vi "xmlParser.vi"(8 "error in (no error)":errorcluster, 10 "XPath Expression":string, 11 "XML File Path":path) -> (0 "error out":errorcluster, 1 "outputArray":string[](array[string]), 2 "outputXML":string, 3 "outputString":string)   [LabVIEW 2018]
uses:
  <vilib>/xml/Close Reference(Node).vi
  <vilib>/xml/NI_XML.lvlib
  <resource>/objmgr/DOMUserDefRef.rc
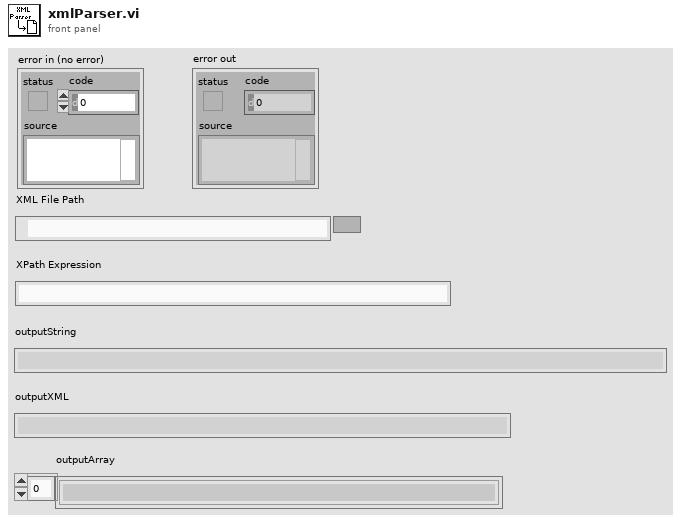
[diagram p1: front panel]
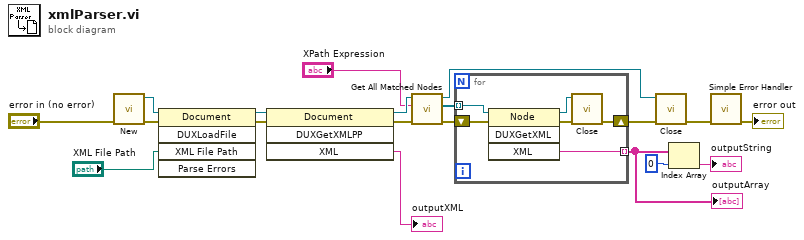
[diagram p0: block diagram]
diagram:
  n1 = call <vilib>:"New.vi"("error in (no error)"="error in (no error)") -> ("error out"=w12:errorcluster, "DOM document out"=w13:refnum<k20>)  [unwired: 7 in]
  n2 = invoke class="Document" method="DUXLoadFile"(reference=w13, error in=w12, "XML File Path"="XML File Path") -> (reference out=w10:refnum<k20>, error out=w11:errorcluster)  [unwired: 2 in, 3 out]
  n3 = invoke class="Document" method="DUXGetXMLPP"(reference=w10, error in=w11) -> (reference out=w14:refnum<k20>, error out=w15:errorcluster, "XML"=→"outputXML":string)  [unwired: 2 in, 1 out]
  n4 = call <vilib>:"Get All Matched Nodes.vi"("error in (no error)"=w15, "XPath expression"="XPath Expression", "node in"=w14) -> ("error out"=w6:errorcluster, "node result array"=w5:refnum<k20>[], "node out"=w8:refnum<k20>)  [unwired: 6 out]
  n5 = for {
    tunnel: w5 -> [w21] mode=indexing
    shift-right: [w23] -> w7
    shift-left: w6 -> [w22]
    tunnel: [w20] -> w16 mode=indexing
    n6 = invoke on="Invoke Node" class="Node" method="DUXGetXML"(reference=w21, error in=w22) -> (reference out=w24:refnum<k20>, error out=w25:errorcluster, "XML"=w20:string)  [unwired: 2 in, 1 out]
    n7 = call-poly <vilib>:"Close.vi"("error in (no error)"=w25, "node"=w24) -> ("error out"=w23:errorcluster)  [unwired: 7 out]
  }
  "outputArray" <- w16
  n8 = call-poly <vilib>:"Close.vi"("error in (no error)"=w7, "node"=w8) -> ("error out"=w9:errorcluster)  [unwired: 7 out]
  n9 = Index Array(array=w16, index=0) -> (element=→"outputString":string)
  n10 = call <vilib>:"Simple Error Handler.vi"("error in (no error)"=w9) -> ("error out"=→"error out":errorcluster)  [unwired: 1 in, 7 out]
